vi "Sweep_device.vi"(8 "error in (no error)":errorcluster, 10 "Message_command":T2, 11 "Command Queue":T3) -> (0 "error out":errorcluster, 2 "dup Message_command":T2, 3 "dup Command Queue":T3)   [LabVIEW 2019]
uses:
  Command_Queue.ctl
  Command_Message.ctl
  Device_List.ctl
panel:
  in  "Device":T1
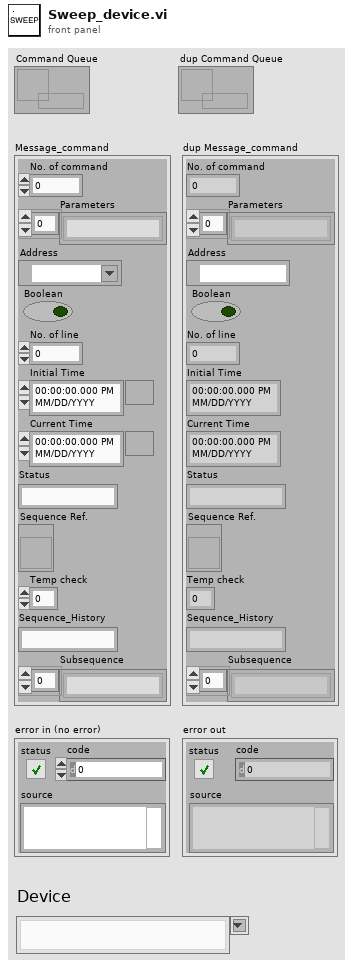
[diagram p1: front panel]
types:
  T1 = typedef "Device_List.ctl" = string
  T2 = typedef "Command_Message.ctl" = cluster{"No. of command":i32, "Parameters":string[], "Address":refnum<visa-resource-name>, "Boolean":bool, "No. of line":i32, "Initial Time":timestamp, "Current Time":timestamp, "Status":string, "Sequence Ref.":refnum<vi>, "Temp check":i32, "Sequence_History":string, "Subsequence":string[]}
  T3 = typedef "Command_Queue.ctl" = refnum<queue>
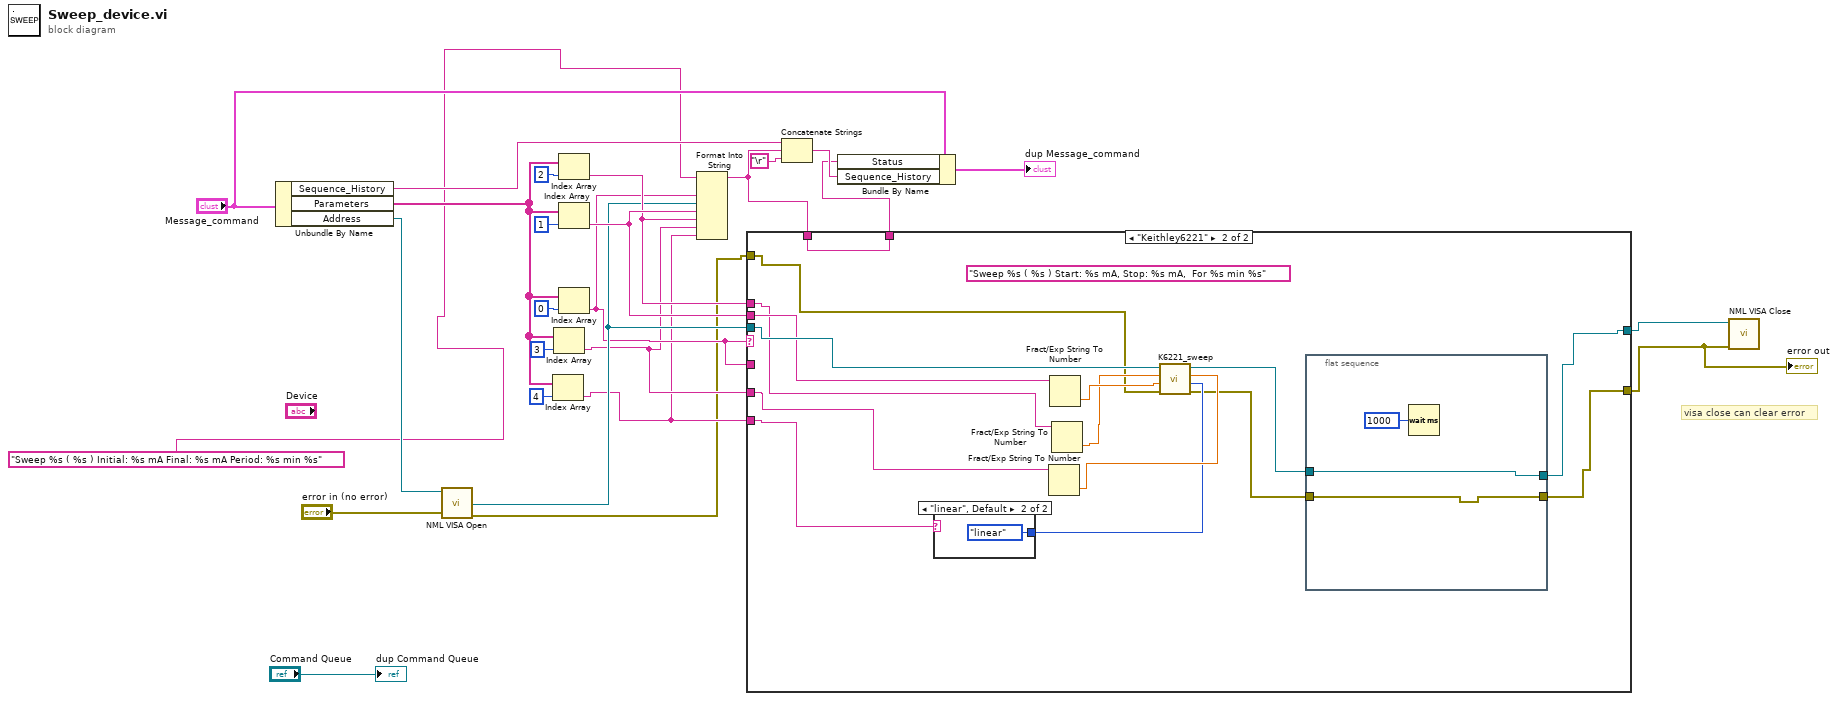
[diagram p0: block diagram]
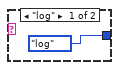
[diagram p3: hidden frame]
diagram:
  # "visa close can clear error"
  n1 = Unbundle By Name("Message_command") -> ("Sequence_History"=w19:string, "Parameters"=w9:string[], "Address"=w13:refnum<visa-resource-name>)
  n2 = call "NML VISA Open.vi"("error in (no error)"="error in (no error)", "VISA resource name"=w13) -> ("error out"=w2:errorcluster, "VISA resource name out"=w15:refnum<visa-resource-name>)  [unwired: 8 in]
  n3 = Index Array(array=w9, index=4) -> (element=w5:string)
  n4 = Index Array(array=w9, index=3) -> (element=w6:string)
  n5 = Index Array(array=w9, index=2) -> (element=w21:string)
  n6 = Index Array(array=w9, index=1) -> (element=w22:string)
  n7 = Index Array(array=w9, index=0) -> (element=w10:string)
  n8 = Format Into String(format string="Sweep %s ( %s ) Initial: %s mA Final: %s mA Period: %s min %s", w10, w15, w22, w21, w6, w5) -> (resulting string=w7:string)  [unwired: 2 in, 1 out]
  n9 = case shown="\"Keithley6221\"" w10 {
    tunnel: w21 -> [_ w38]
    tunnel: w22 -> [_ w39]
    tunnel: w15 -> [w28 w44]
    tunnel: w2 -> [w29 w34]
    tunnel: [w29 w33] -> w1
    tunnel: [w28 w31] -> w14
    tunnel: w7 -> [w27 w35]
    tunnel: [w27 w35] -> w8
    tunnel: w10 -> [_ _]
    tunnel: w6 -> [_ w37]
    tunnel: w5 -> [_ w36]
    frame "False", Default {
    }
    frame "Keithley6221" {
      (unwired) "Sweep %s ( %s ) Start: %s mA, Stop: %s mA,  For %s min %s" ("format string")
      n10 = case shown="\"linear\", Default" w36 {
        tunnel: [enum16{"linear", "log", "custom"}."log" ("Enum") enum16{"linear", "log", "custom"}."linear" ("Enum")] -> w40
        frame "log" {
        }
        frame "linear", Default {
        }
      }
      n11 = Fract/Exp String To Number(string=w37) -> (number=w41:dbl)  [unwired: 3 in, 1 out]
      n12 = Fract/Exp String To Number(string=w39) -> (number=w43:dbl)  [unwired: 3 in, 1 out]
      n13 = Fract/Exp String To Number(string=w38) -> (number=w42:dbl)  [unwired: 3 in, 1 out]
      n14 = call "K6221_sweep.vi"("VISA resource name"=w44, "Stop mA"=w42, "Start mA"=w43, "error in"=w34, "Time min"=w41, "mode"=w40) -> ("VISA resource name 2"=w30:refnum<visa-resource-name>, "error out"=w32:errorcluster)  [unwired: 1 in]
      n15 = flat-sequence {
        tunnel: [w47] -> w33
        tunnel: w32 -> [w47]
        tunnel: [w46] -> w31
        tunnel: w30 -> [w46]
        frame #0 {
          n16 = Wait (ms)(milliseconds to wait=u32 1000) -> ()  [unwired: 1 out]
        }
      }
    }
  }
  "error out" <- w1
  n17 = Concatenate Strings(w19, w7, "\r") -> (w17:string)
  n18 = Bundle By Name(cluster="Message_command", "Status"=w8, "Sequence_History"=w17) -> (→"dup Message_command":T2)
  n19 = call "NML VISA Close.vi"("Error In"=w1, "VISA resource name"=w14) -> ()  [unwired: 9 in, 1 out]
  "dup Command Queue" <- "Command Queue"
